vi "FinalReportResult.vi"(5 "TXID":string="6444", 7 "RXID":string="6445", 9 "BOUNCEID":string="1491", 11 "error in (no error)":errorcluster, 13 "Run Final Report (T)":bool=TRUE) -> (1 "standard output":string="rxId:6445\r\ntxId:6444\r\nbid:1491\r\nOverall Status:  PASS\r\nSerial Number: RA23070129\r\nReceive Power Supply Consumption Limits : Pass\r\nReceiver Input Frequency : Pass\r\nReceiver Gain : Pass\r\nReceiver Noise Figure : Pass\r\nTransmit Output Frequency : Pass\r\nTransmit Power Supply Consumption Limits : Pass\r\nTransmit In-Band Output Peak Power : Pass\r\nHarmonics : Pass\r\nReference Source Port Return Loss : Pass\r\nTransmit Power Flatness : Pass\r\nTemperature Sensors : Pass\r\nBounce Test : Pass", 2 "result(ary)":string[](array[string])=["Overall Status:  PASS", "Serial Number: RA23070129", "Receive Power Supply Consumption Limits : Pass", "Receiver Input Frequency : Pass", "Receiver Gain : Pass", "Receiver Noise Figure : Pass", "Transmit Output Frequency : Pass", "Transmit Power Supply Consumption Limits : Pass", "Transmit In-Band Output Peak Power : Pass", "Harmonics : Pass", "Reference Source Port Return Loss : Pass", "Transmit Power Flatness : Pass", "Temperature Sensors : Pass", "Bounce Test : Pass"], 3 "pass?(t)":bool=TRUE, 6 "report_script_err?(t)":bool, 15 "error out":errorcluster)   [LabVIEW 2018]
uses:
  Initialize References/Sequence Globals.vi
panel:
  out "py dir (path)":path
  out "Flag sid?(t)":bool
  out "IdMessage":string="One of the id's is NOT valid number between 1 - 99999" caption="Message"
  out "InvalidData?(t)":bool caption="OK"
  out "Numeric":i32
  out "Version":string="3500007  2.0.0"
  out "index of element":i32=3
  out "RESULT (P/F)":string="PASS"
  out "standard error":string
  out "DUT S/N":string="RA23070129"
  out ".ini file(data)":string="[PartNumber]\nleidos = AX0125-35614-00\n\n[SWRevision]\npmic = Rev 1.1\ntestboard = Rev 8c61\n\n[Testname]\ntest = ATP\n\n[Report]\ntitle = Wideband Antenna Module\n\n[LetterHead]\npath = rageletterhead.png\n\n[TableNames]\ncond_table = TEST CONDITIONS FOR PRODUCTION\nresult_table_name = TEST RESULTS FOR ANTENNA WIDEBAND ANTENNA MODULE\n\n[Address]\nstreet_Suite = 175 Cabot St, Suite 315\ncity_state_zip = Lowell, MA, 01854\nphone = Phone : (978) 941-4900\nwebsite = Website : https:www.ragesystems.com\n\n[TestLimits]\ngainHigh = 60\ngainLow = 30\n\nnoiseFigure_band = 16\n\npowerCon = 12\nreturnLoss = -5\nflatLim = 8\ntxPoutLow = 6\ntxPouthigh = 6\ntemp_low   = -99\nnoise_figure_filter = -1\nh2_lim = -15\nhx_lim = -10\nfreq_start_tx = 20\nfreq_end_tx = 35\n\nfreq_start_rx = 20\nfreq_end_rx = 35\n\ngainlow = 6.5\ngainhigh = 6.5\n\ntxPout_u = 0\ntxPout_l = -20\n\nfreq_start_flat = 20\nfreq_end_flat = 35\n\nfreq_start_nf = 20\nfreq_end_nf  = 40\nnf_20_40_GHz = 22\n\ntxhigh  = 107\ntxlow  = 94\nslope = 2.75\n\n[BouncePowerLimits]\nupper = 2\nlower = -12\n[BounceFreqRange]\nupper = -6\nlower = -6.5\n"
  # "6443\t6444\t6445\t1491"
  # "Process the result of Tetra WAM rev_C final test files"
  # "Input Data From Post Processer"
  # "Result"
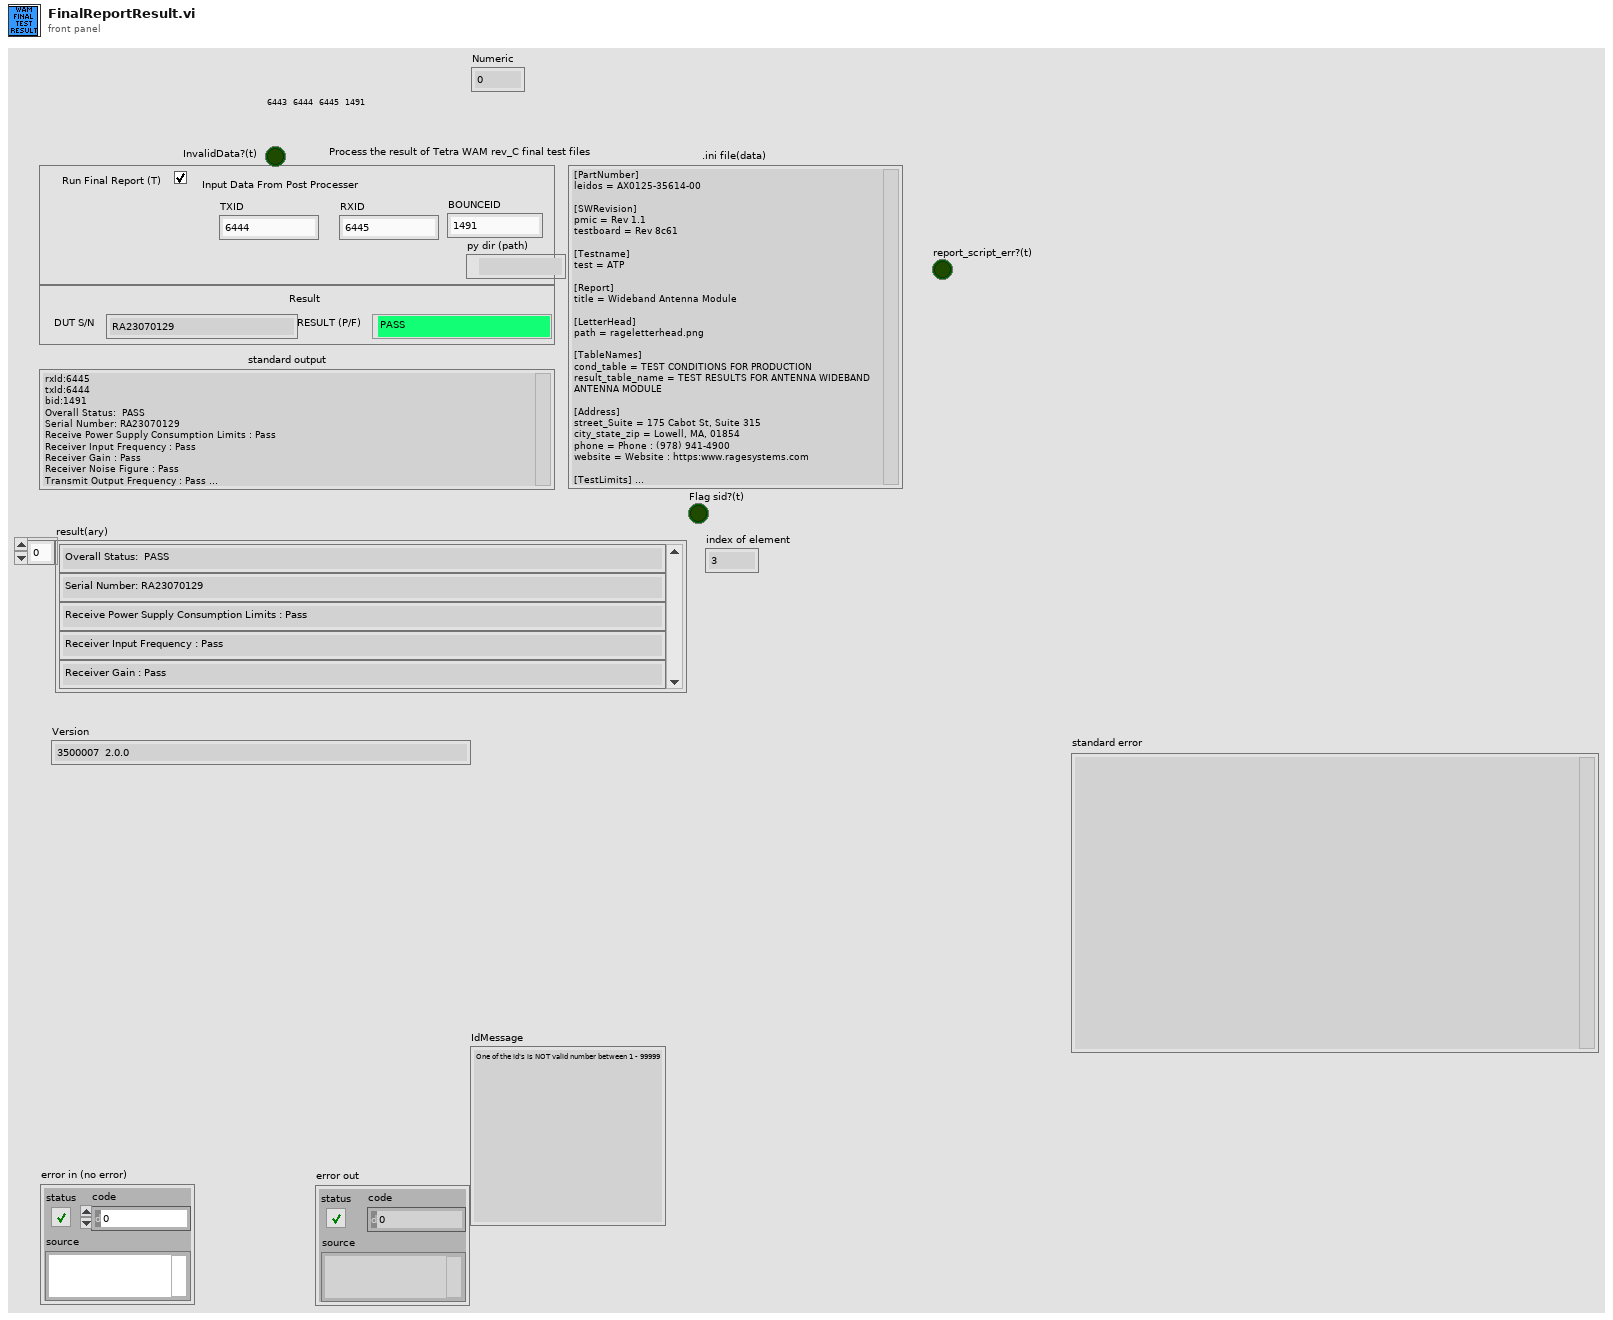
[diagram p1: front panel]
types:
  T1 = enum16{"Left Button", "Center Button", "Right Button", "Window Close"}
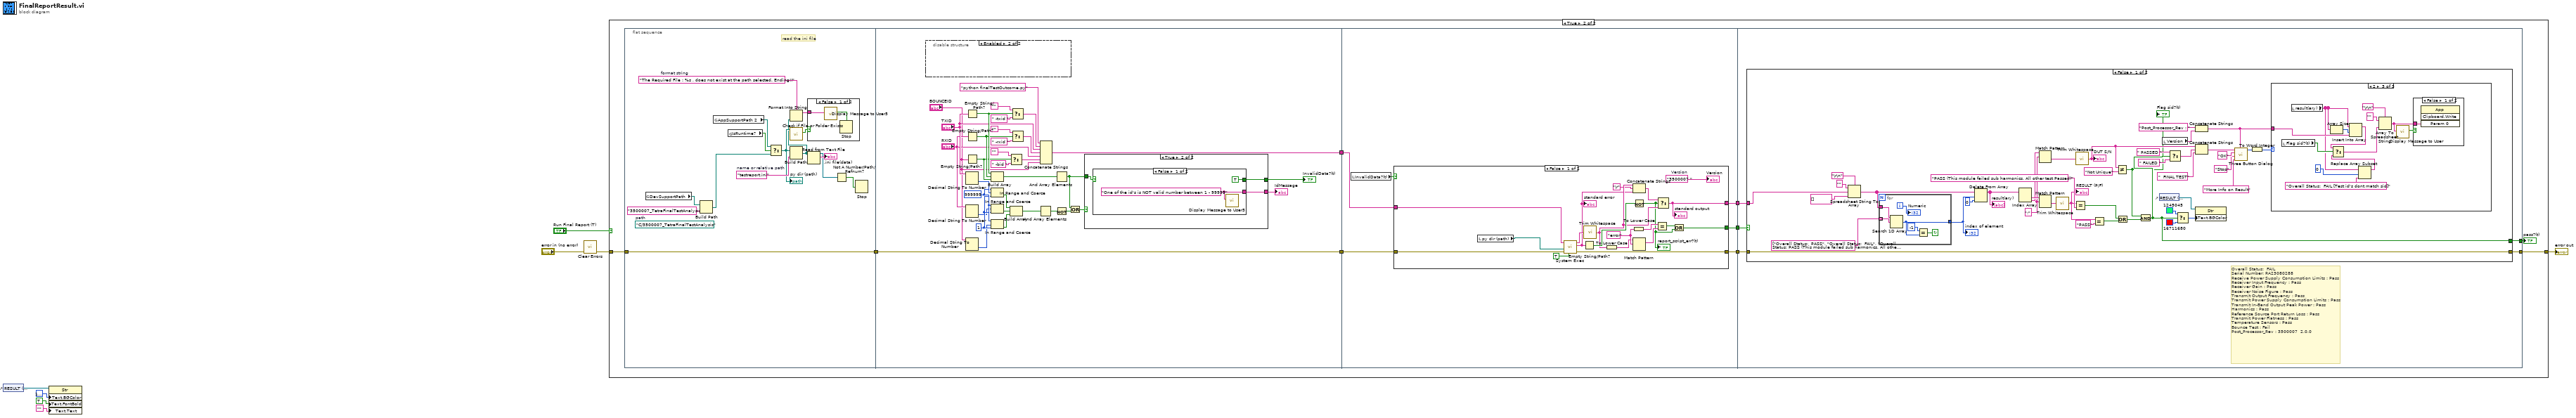
[diagram p0: block diagram]
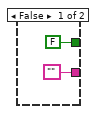
[diagram p4: hidden frame]
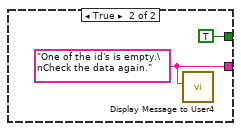
[diagram p5: hidden frame]
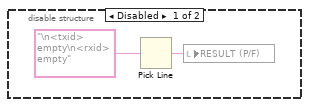
[diagram p6: hidden frame]
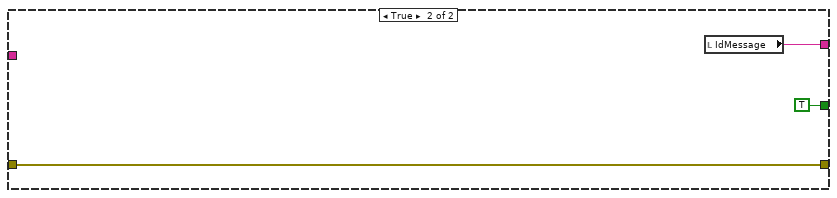
[diagram p7: hidden frame]
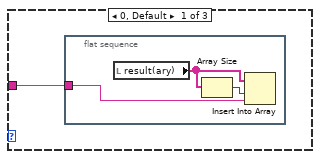
[diagram p8: hidden frame]
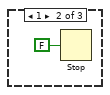
[diagram p9: hidden frame]
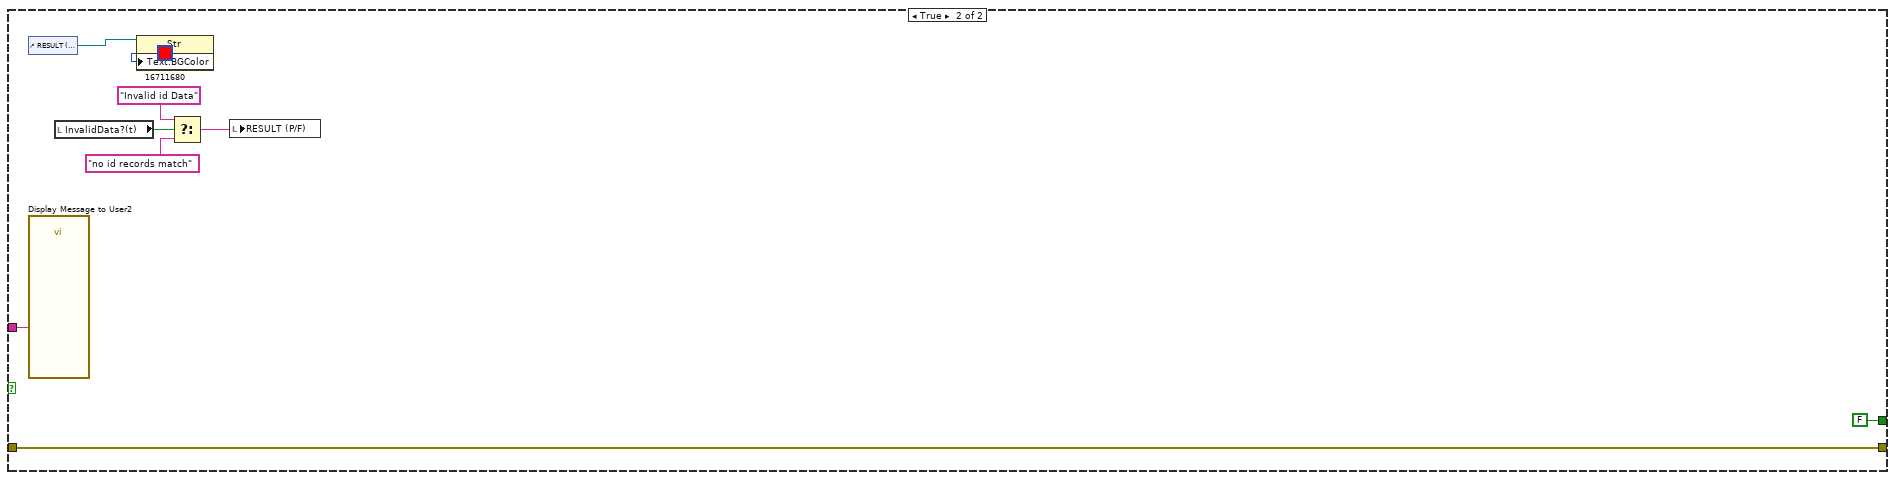
[diagram p11: hidden frame]
diagram:
  n1 = control-ref of="RESULT (P/F)"() -> (w5:refnum<vi>)
  n2 = property class="Str"(reference=w5, "Text.BGColor"=u32 16777216, "Text.FontBold"=TRUE ("Text.Font:Bold"), "Text.Text"="") -> ()  [unwired: 1 in, 2 out]
  n3 = call <vilib>:"Clear Errors.vi"("error in (no error)"="error in (no error)") -> ("error out"=w1:errorcluster)  [unwired: 5 in, 1 out]
  n4 = case shown="True" "Run Final Report (T)" {
    tunnel: w1 -> [w9 w14]
    tunnel: [w9 w13] -> w7
    frame False {
    }
    frame True {
      n5 = flat-sequence {
        tunnel: [w33] -> w18
        tunnel: w14 -> [w33]
        tunnel: [w68] -> w17
        tunnel: [w58] -> w16
        tunnel: w18 -> [w58]
        tunnel: w17 -> [w86]
        tunnel: [w85] -> w15
        tunnel: w16 -> [w84]
        tunnel: [w83] -> w12
        tunnel: [w82] -> w10
        tunnel: w15 -> [w111]
        tunnel: [w112] -> w13
        tunnel: w12 -> [w113]
        tunnel: [w110] -> w11
        tunnel: w10 -> [w114]
        frame #0 {
          w27 = "The Required File : %s , does not exist at the path selected. Ending!!"  # format string
          (unwired) path "C:/3500007_TetraFinalTestAnalysis"  # path
          w31 = "testreport.ini"  # name or relative path
          # "read the ini file"
          n6 = global read "Sequence Globals.vi" "DevSupportPath"() -> (w21:path)
          n7 = Build Path(base path=w21, name or relative path="3500007_TetraFinalTestAnalysis") -> (appended path=w19:path)
          n8 = global read "Sequence Globals.vi" "AppSupportPath 2"() -> (w29:path)
          n9 = global read "Sequence Globals.vi" "IsRuntime?"() -> (w30:bool)
          n10 = Select(t=w29, s=w30, f=w19) -> (s? t:f=w25:path)
          "py dir (path)" <- w25
          n11 = call <vilib>:"Check if File or Folder Exists.vi"("path"=w25) -> ("file or folder exists?"=w28:bool)  [unwired: 8 in, 2 out]
          n12 = Build Path(base path=w25, name or relative path=w31) -> (appended path=w22:path)
          n13 = Format Into String(format string=w27, w22) -> (resulting string=w26:string)  [unwired: 2 in, 1 out]
          n14 = case shown="False" w28 {
            tunnel: w26 -> [w35 _]
            frame False {
              n15 = call "Display Message to User5"("Message"=w35) -> ("OK"=w34:bool)  [unwired: 9 in, 1 out]
              n16 = Stop(stop? (T)=w34) -> ()
            }
            frame True {
            }
          }
          n17 = Read from Text File(file (use dialog)=w22) -> (refnum out=w24:refnum<file>, text=→".ini file(data)":string)  [unwired: 3 in, 2 out]
          n18 = Not A Number/Path/Refnum?(number/path/refnum=w24) -> (NaN/Path/Refnum?=w23:bool)
          n19 = Stop(stop? (T)=w23) -> ()
        }
        frame #1 {
          w44 = 1 ("lower limit")
          w45 = 999999 ("upper limit")
          n20 = disable-structure shown="Enabled" {
            frame Disabled {
              n21 = Pick Line(multi-line string="\n<txid> empty\n<rxid> empty") -> (output string=w79:string)  [unwired: 2 in]
              n22 = local write "RESULT (P/F)"(w79) -> ()
            }
            frame Enabled {
            }
          }
          n23 = Decimal String To Number(string="TXID") -> (number=w46:i32)  [unwired: 2 in, 1 out]
          n24 = Decimal String To Number(string="RXID") -> (number=w43:i32)  [unwired: 2 in, 1 out]
          n25 = Decimal String To Number(string="BOUNCEID") -> (number=w42:i32)  [unwired: 2 in, 1 out]
          n26 = Empty String/Path?(string/path="TXID") -> (empty?=w53:bool)
          n27 = Empty String/Path?(string/path="RXID") -> (empty?=w52:bool)
          n28 = Empty String/Path?(string/path="BOUNCEID") -> (empty?=w51:bool)
          n29 = Build Array(w53, w52, w51) -> (w37:bool[])
          n30 = In Range and Coerce(upper limit=w45, x=w46, lower limit=w44) -> (In Range?=w56:bool)  [unwired: 1 out]
          n31 = In Range and Coerce(upper limit=w45, x=w43, lower limit=w44) -> (In Range?=w55:bool)  [unwired: 1 out]
          n32 = In Range and Coerce(upper limit=w45, x=w42, lower limit=w44) -> (In Range?=w54:bool)  [unwired: 1 out]
          n33 = Select(t="", s=w51, f=" -bid " ("string")) -> (s? t:f=w66:string)
          n34 = Build Array(w56, w55, w54) -> (w57:bool[])
          n35 = Select(t="", s=w53, f=" -txid " ("string")) -> (s? t:f=w61:string)
          n36 = Select(t="", s=w52, f=" -rxid " ("string")) -> (s? t:f=w63:string)
          n37 = And Array Elements(Boolean array=w57) -> (logical AND=w38:bool)
          n38 = Concatenate Strings("python finalTestOutcome.py" ("command line"), w61, "TXID", w63, "RXID", w66, "BOUNCEID") -> (w68:string)
          n39 = And Array Elements(Boolean array=w37) -> (logical AND=w40:bool)
          n40 = Not(x=w38) -> (.not. x?=w36:bool)
          n41 = Or(x=w40, y=w36) -> (x .or. y?=w41:bool)
          n42 = case shown="True" w41 {
            tunnel: [FALSE ("OK") w74] -> w50
            tunnel: w40 -> [_ w73]
            tunnel: ["" w72] -> w39
            frame False {
            }
            frame True {
              n43 = case shown="False" w73 {
                tunnel: [TRUE ("OK") TRUE ("OK")] -> w74
                tunnel: [w75 w77] -> w72
                frame False {
                  w75 = "One of the id's is NOT valid number between 1 - 99999" ("Message")
                  n44 = call "Display Message to User3"("Message"=w75) -> ()  [unwired: 9 in, 2 out]
                }
                frame True {
                  w77 = "One of the id's is empty.\nCheck the data again." ("Message")
                  n45 = call "Display Message to User4"("Message"=w77) -> ()  [unwired: 9 in, 2 out]
                }
              }
            }
          }
          "InvalidData?(t)" <- w50
          "IdMessage" <- w39
        }
        frame #2 {
          n46 = local read "InvalidData?(t)"() -> (w81:bool)
          n47 = case shown="False" w81 {
            tunnel: w86 -> [w105 _]
            tunnel: [w104 w107] -> w85
            tunnel: w84 -> [w102 w107]
            tunnel: [w92 TRUE] -> w83
            tunnel: [w89 w109] -> w82
            frame False {
              w88 = "3500007 "  # Version
              w100 = "error" ("regular expression")
              n48 = local read "py dir (path)"() -> (w87:path)
              n49 = call <vilib>:"System Exec.vi"("run minimized? (F)"=TRUE, "error in (no error)"=w102, "working directory"=w87, "command line"=w105) -> ("error out"=w104:errorcluster, "standard error"=w91:string, "standard output"=w103:string)  [unwired: 4 in, 1 out]
              "standard error" <- w91
              n50 = Empty String/Path?(string/path=w91) -> (empty?=w96:bool)
              n51 = call <vilib>:"Trim Whitespace.vi"("string"=w103) -> ("trimmed string"=w95:string)  [unwired: 1 in]
              n52 = To Lower Case(string=w95) -> (all lower case string=w98:string)
              n53 = To Lower Case(string=w100) -> (all lower case string=w99:string)
              n54 = Concatenate Strings(w95, "\r", w91) -> (w93:string)
              n55 = Match Pattern(string=w98, regular expression=w100) -> (match substring=w101:string)  [unwired: 1 in, 3 out]
              n56 = Not(x=w96) -> (.not. x?=w90:bool)
              "report_script_err?(t)" <- w90
              n57 = Equal?(x=w99, y=w101) -> (x = y?=w97:bool)
              n58 = Select(t=w93, s=w90, f=w95) -> (s? t:f=w89:string)
              "standard output" <- w89
              n59 = Or(x=w97, y=w90) -> (x .or. y?=w92:bool)
              "Version" <- w88
            }
            frame True {
              n60 = local read "IdMessage"() -> (w109:string)
            }
          }
        }
        frame #3 {
          # "Overall Status:  FAIL\nSerial Number: RA23080288\nReceive Power Supply Consumption Limits : Pass\nReceiver Input Frequency : Pass\nReceiver Gain : Pass\nReceiver Noise Figure : Pass\nTransmit Output Frequency : Pass\nTransmit Power Supply Consumption Limits : Pass\nTransmit In-Band Output Peak Power : Pass\nHarmonics : Pass\nReference Source Port Return Loss : Pass\nTransmit Power Flatness : Pass\nTemperature Sensors : Pass\nBounce Test : Fail\nPost_Processor_Rev : 3500007  2.0.0"
          n61 = case shown="False" w113 {
            tunnel: w114 -> [w153 w190]
            tunnel: [w131 w184] -> w112
            tunnel: w111 -> [w131 w184]
            tunnel: [w117 FALSE] -> w110
            frame False {
              w149 = ":" ("regular expression")
              n62 = Spreadsheet String To Array(delimiter (Tab)="\r\n", format string="", spreadsheet string=w153, array type (2D Dbl)=string[] []) -> (array=w130:string[])
              n63 = for {
                tunnel: w130 -> [w162]
                tunnel: string[] ["Overall Status:  PASS", "Overall Status:  FAIL", "Overall Status: PASS (This module failed sub harmonics. All other test Passed)"] ("array type (2D Dbl)") -> [w158] mode=indexing
                tunnel: [w161] -> w129
                i -> [w157]
                stop <- w159 continue-if-true
                n64 = Search 1D Array(1D array=w162, element=w158) -> (index of element=w161:i32)  [unwired: 1 in]
                n65 = Equal?(x=-1, y=w161) -> (x = y?=w159:bool)
                "Numeric" <- w157
              }
              "index of element" <- w129
              n66 = Delete From Array(array=w130, length=w129, index=0) -> (array with subset deleted=w128:string[])  [unwired: 1 out]
              "result(ary)" <- w128
              n67 = Index Array(array=w128) -> (element #1=w151:string, element #2=w150:string)  [unwired: 2 in]
              n68 = Match Pattern(string=w150, regular expression=w149) -> (after substring=w148:string)  [unwired: 1 in, 3 out]
              n69 = Match Pattern(string=w151, regular expression=w149) -> (after substring=w147:string)  [unwired: 1 in, 3 out]
              n70 = call <vilib>:"Trim Whitespace.vi"("string"=w147) -> ("trimmed string"=w123:string)  [unwired: 1 in]
              "RESULT (P/F)" <- w123
              n71 = Equal?(x=w123, y="PASS (This module failed sub harmonics. All other test Passed)") -> (x = y?=w122:bool)
              n72 = call <vilib>:"Trim Whitespace.vi"("string"=w148) -> ("trimmed string"=w119:string)  [unwired: 1 in]
              "DUT S/N" <- w119
              n73 = Equal?(x=w123, y="PASS") -> (x = y?=w121:bool)
              n74 = Not Equal?(x=w119, y="Not Unique") -> (x != y?=w116:bool)
              "Flag sid?(t)" <- w116
              n75 = Or(x=w122, y=w121) -> (x .or. y?=w120:bool)
              n76 = And(x=w116, y=w120) -> (x .and. y?=w117:bool)
              n77 = control-ref of="RESULT (P/F)"() -> (w140:refnum<vi>)
              n78 = local read "Version"() -> (w127:string)
              n79 = Select(t=" PASSED " ("y"), s=w117, f=" FAILED " ("y")) -> (s? t:f=w144:string)
              n80 = Select(t=u32 1245045, s=w117, f=u32 16711680) -> (s? t:f=w141:u32)
              n81 = Concatenate Strings("Post_Processor_Rev : " ("string"), w127) -> (w126:string)
              n82 = Concatenate Strings(w119, w144, "  FINAL TEST" ("string")) -> (w137:string)
              n83 = property class="Str"(reference=w140, "Text.BGColor"=w141) -> ()  [unwired: 1 in, 2 out]
              n84 = call <vilib>:"Three Button Dialog.vi"("Window Title (\"\")"=w126, "Right Button Text (\"Cancel\")"="More Info on Result" ("Right Button Text (\"Cancel\")"), "Center Button Text (\"No\")"="Stop" ("Center Button Text (\"No\")"), "Left Button Text (\"Yes\")"="OK" ("Left Button Text (\"Yes\")"), "message"=w137) -> ("Which Button?"=w133:T1)  [unwired: 6 in]
              n85 = To Word Integer(number=w133) -> (16bit integer=w132:i16)
              n86 = case shown="2" w132 {
                tunnel: w126 -> [w163 _ w176]
                frame 0, Default {
                  n87 = flat-sequence {
                    tunnel: w163 -> [w165]
                    frame #0 {
                      n88 = local read "result(ary)"() -> (w166:string[])
                      n89 = Array Size(array=w166) -> (size(s)=w164:i32)
                      n90 = Insert Into Array(array=w166, index=w164, new element=w165) -> ()  [unwired: 1 out]
                    }
                  }
                }
                frame 1 {
                  n91 = Stop(stop? (T)=FALSE) -> ()
                }
                frame 2 {
                  n92 = local read "Flag sid?(t)"() -> (w173:bool)
                  n93 = local read "result(ary)"() -> (w171:string[])
                  n94 = Array Size(array=w171) -> (size(s)=w175:i32)
                  n95 = Insert Into Array(array=w171, index=w175, new element=w176) -> (w172:string[])
                  n96 = Replace Array Subset(array=w171, new element="Overall Status:  FAIL [Test id's dont match sid]", index=0) -> (w168:string[])
                  n97 = Select(t=w172, s=w173, f=w168) -> (s? t:f=w174:string[])
                  n98 = Array To Spreadsheet String(delimiter (Tab)="\r\n", array=w174, 3:"" ("format string")) -> (spreadsheet string=w179:string)
                  n99 = call "Display Message to User"("Message"=w179) -> ("OK"=w180:bool)  [unwired: 9 in, 1 out]
                  n100 = case shown="False" w180 {
                    tunnel: w179 -> [w181 _]
                    frame False {
                      n101 = invoke class="App" method="Clipboard.Write"("Param 0"=w181) -> ()  [unwired: 3 in, 4 out]
                    }
                    frame True {
                    }
                  }
                }
              }
            }
            frame True {
              n102 = control-ref of="RESULT (P/F)"() -> (w183:refnum<vi>)
              n103 = call "Display Message to User2"("Message"=w190) -> ()  [unwired: 9 in, 2 out]
              n104 = local read "InvalidData?(t)"() -> (w188:bool)
              n105 = property class="Str"(reference=w183, "Text.BGColor"=u32 16711680) -> ()  [unwired: 1 in, 2 out]
              n106 = Select(t="Invalid id Data", s=w188, f="no id records match" ("RESULT (P/F)")) -> (s? t:f=w186:string)
              n107 = local write "RESULT (P/F)"(w186) -> ()
            }
          }
        }
      }
      "pass?(t)" <- w11
    }
  }
  "error out" <- w7
